vi "draw_field.vi"(0 "Field_Astrometry":T2 {"NAXIS" format="%#.6g"}, 1 "FOV":dbl, 2 "NaxisMax":dbl=1000000.0, 3 "Ring":u16(ring) items=["Square", "Circle"], 5 "Table_Astrometry":T2 {"CRPIX" format="%.1f"}, 6 "Rotation effective":dbl, 9 "Ues Constant Size ?":bool, 11 "margin/size":dbl=5.0, 12 "MirrorAvatar":T1={"Empreinte du miroir [arcmin]"=12.075, "Cur X"=-5.0, "Cur Y"=35.0, "Vignetting du miroir [armin]"=17.764, "FOV du miroir [arcmin]"=12.075, "LimXPesto"=-5.0, "BrasPesto"=FALSE}) -> (4 "TableXYPos":cluster{dbl[], dbl[]}[](graph), 10 "X Scale.Range":T3, 13 "ImgDEC":dbl format="%.6f", 14 "ImgRA":dbl format="%.6f", 15 "Y Scale.Range":T3)   [LabVIEW 2019]
uses:
  <vilib>/Utility/miscctls.llb/LVRangeTypeDef.ctl
  <vilib>/Analysis/coordinate.llb/2D Cartesian Coordinate Rotation (Array).vi
  <vilib>/Analysis/baseanly.llb/Mean (DBL).vi
  <vilib>/Analysis/NI_AALPro.lvlib
  <vilib>/Analysis/NI_AALBase.lvlib
panel:
  out "Rotation effective (rad)":dbl
  out "Vig Y":dbl[](array[numeric])
  out "Vig X":dbl[](array[numeric])
  in  "RayondeVignetting [arcmin]":dbl=50.0
  out "Y_arr":dbl[](array[numeric])
  out "X_arr":dbl[](array[numeric])
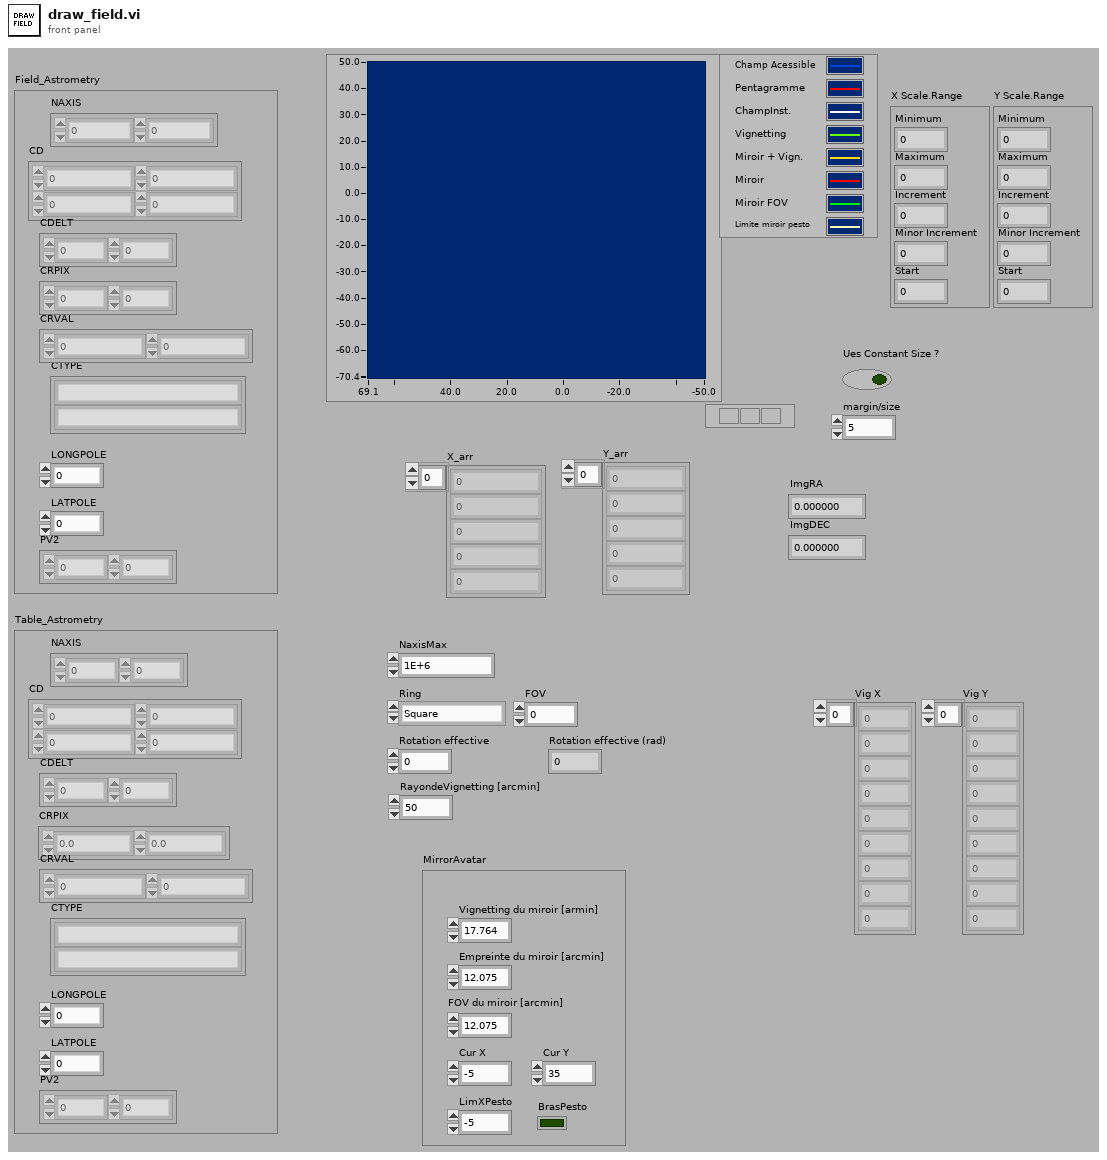
[diagram p1: front panel]
types:
  T1 = cluster{"Empreinte du miroir [arcmin]":dbl, "Cur X":dbl, "Cur Y":dbl, "Vignetting du miroir [armin]":dbl, "FOV du miroir [arcmin]":dbl, "LimXPesto":dbl, "BrasPesto":bool}
  T2 = cluster{"NAXIS":dbl[], "CD":dbl[][], "CDELT":dbl[], "CRPIX":dbl[], "CTYPE":string[], "CRVAL":dbl[], "LONGPOLE":dbl, "LATPOLE":dbl, "PV2":dbl[]}
  T3 = typedef "LVRangeTypeDef.ctl" = cluster{"Minimum":dbl, "Maximum":dbl, "Increment":dbl, "Minor Increment":dbl, "Start":dbl}
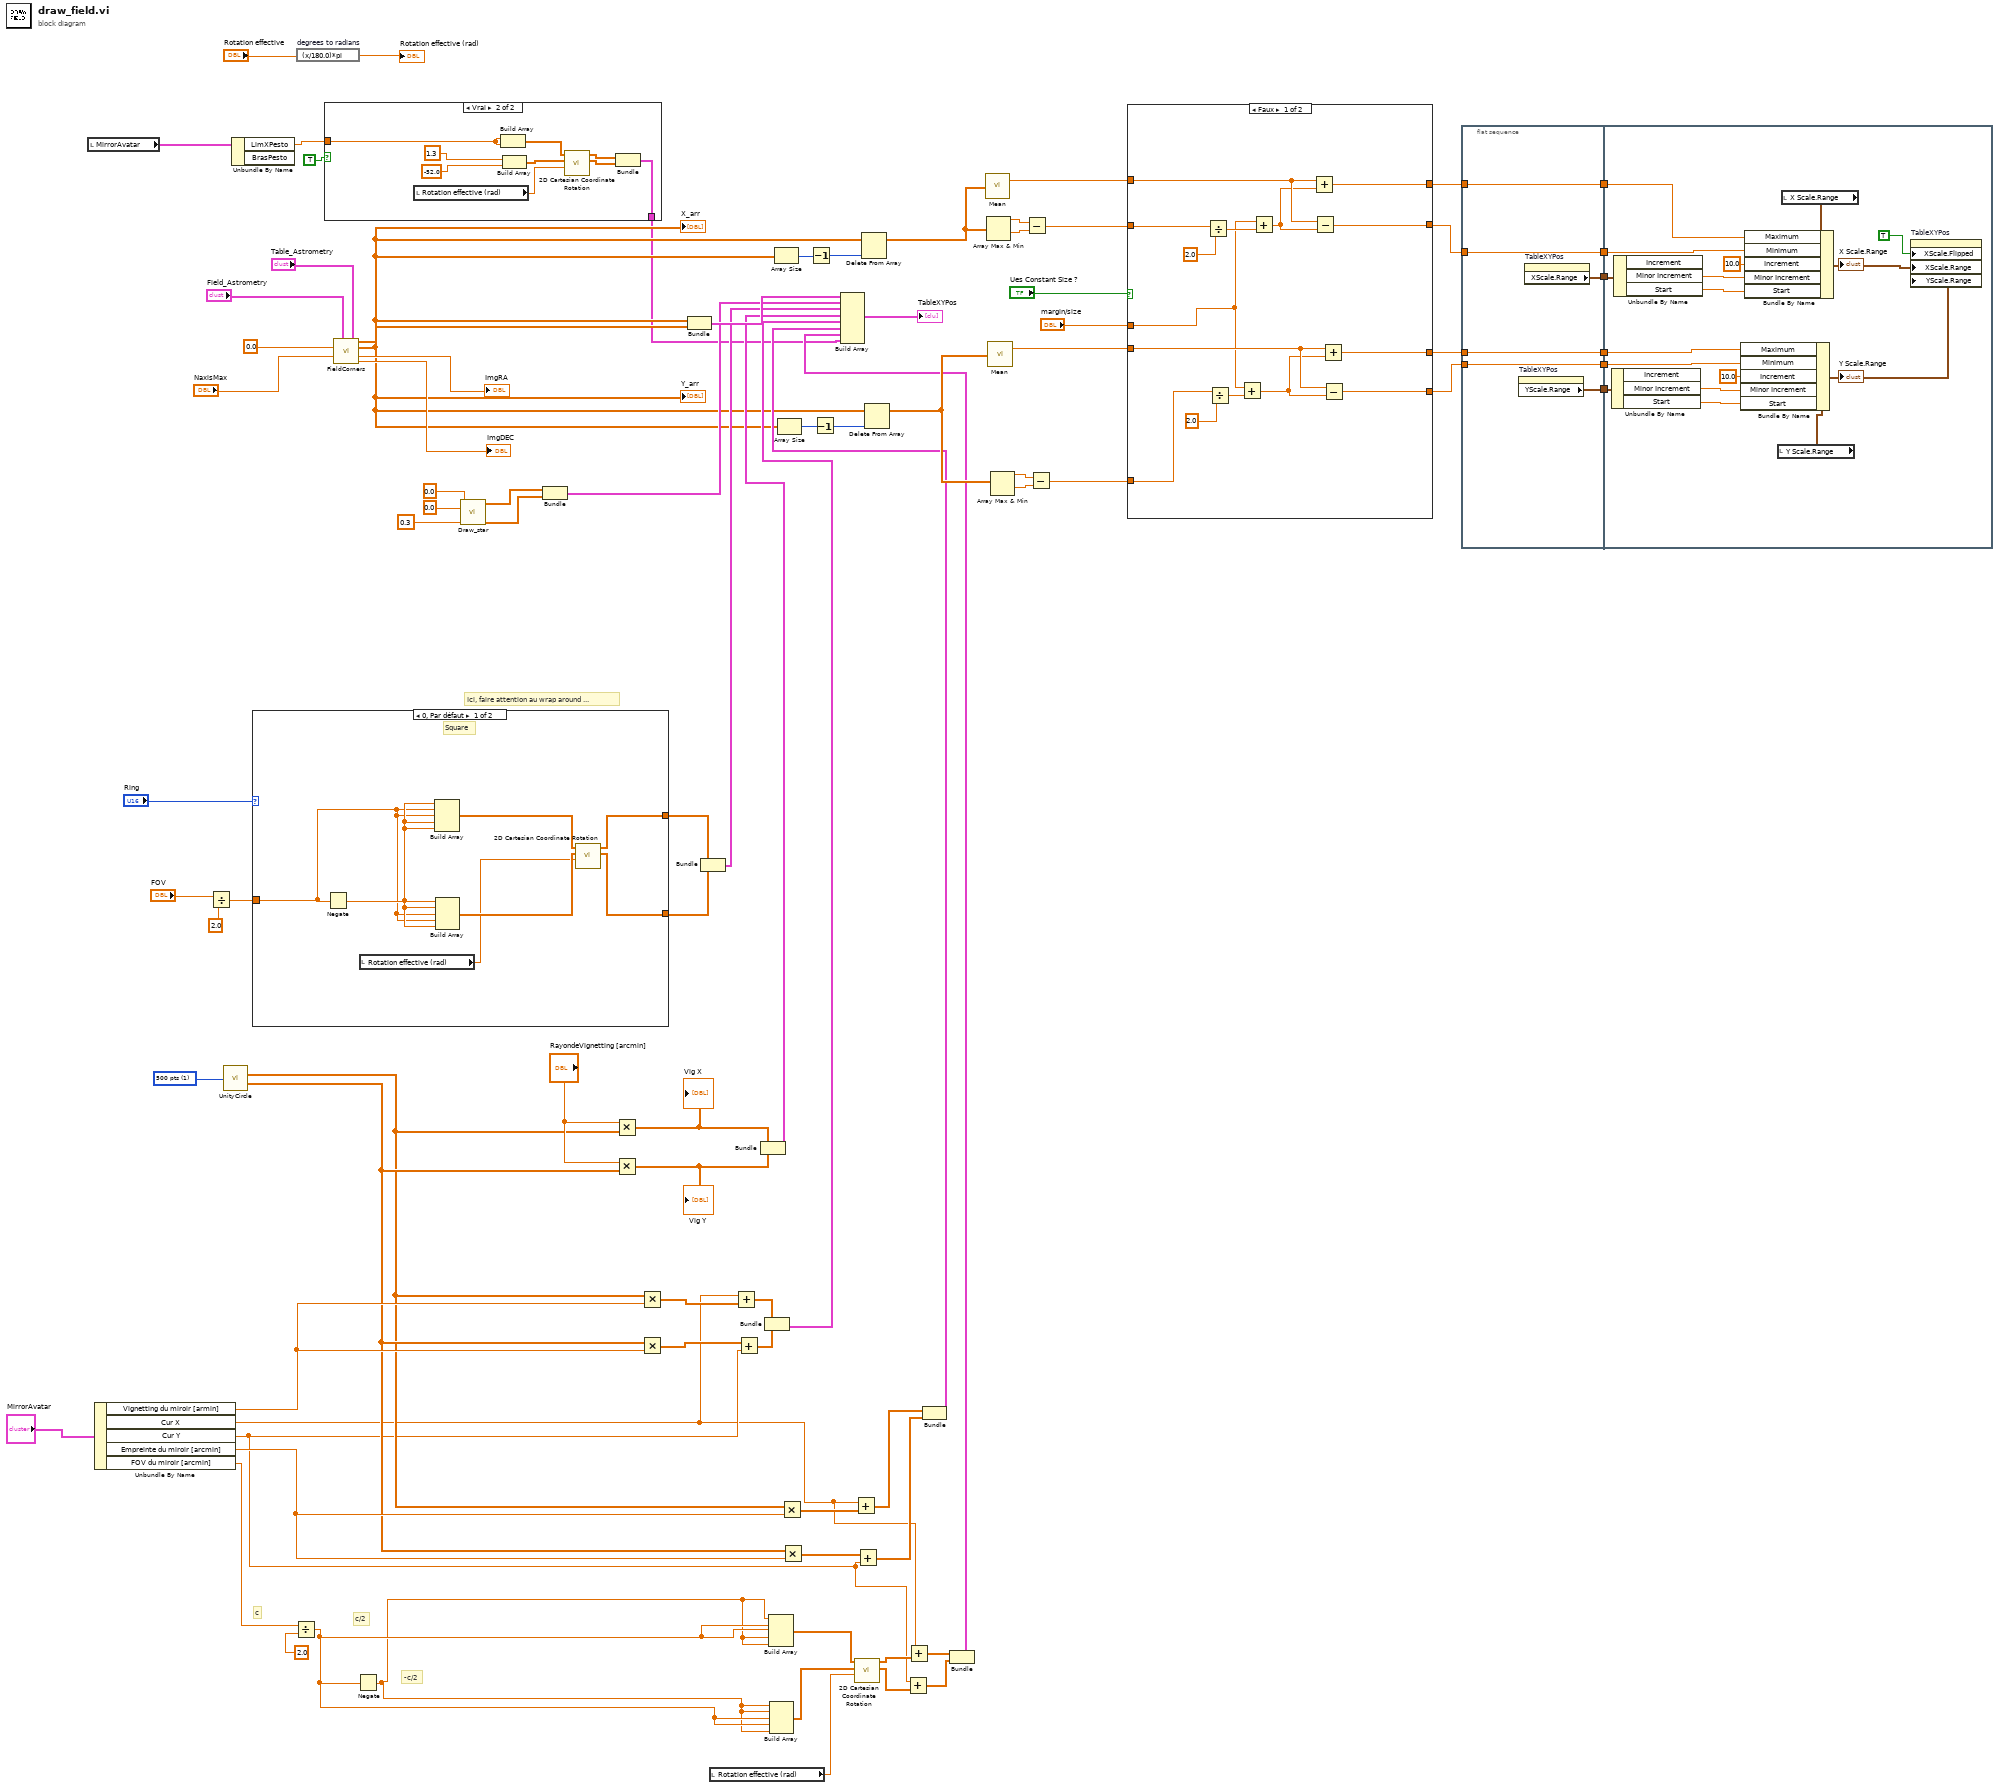
[diagram p0: block diagram]
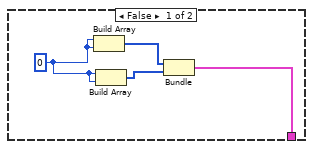
[diagram p2: hidden frame]
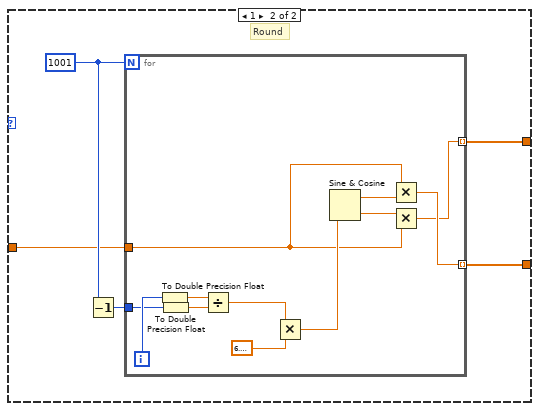
[diagram p3: hidden frame]
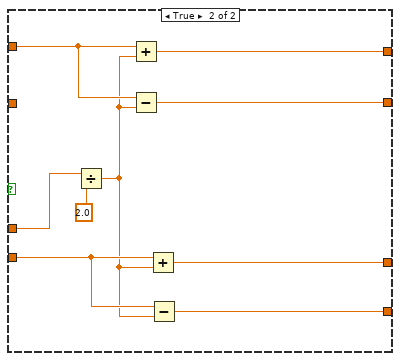
[diagram p4: hidden frame]
diagram:
  w30 = u16 1 items=["100 pts", "500 pts", "1000 pts"] ("Ring")
  # "c"
  # "c/2"
  # "-c/2"
  # "Ici, faire attention au wrap around ..."
  n1 = local read "MirrorAvatar"() -> (w3:T1)
  n2 = Unbundle By Name("MirrorAvatar") -> ("Vignetting du miroir [armin]"=w26:dbl, "Cur X"=w6:dbl, "Cur Y"=w7:dbl, "Empreinte du miroir [arcmin]"=w25:dbl, "FOV du miroir [arcmin]"=w21:dbl)
  n3 = Divide(x="FOV", y=2.0) -> (x/y=w60:dbl)
  n4 = call "UnityCircle.vi"("Ring"=w30) -> ("Circle X"=w23:dbl[], "Circle Y"=w24:dbl[])  [unwired: 13 in]
  n5 = Unbundle By Name(w3) -> ("LimXPesto"=w2:dbl)  [unwired: 1 out]
  n6 = case shown="0, Par défaut" "Ring" {
    tunnel: w60 -> [w95 w99]
    tunnel: [w91 w97] -> w65
    tunnel: [w90 w98] -> w64
    frame 0, Default {
      # "Square"
      n7 = Negate(x=w95) -> (-x=w96:dbl)
      n8 = local read "Rotation effective (rad)"() -> (w92:dbl)
      n9 = Build Array(w96, w95, w95, w96, w96) -> (w94:dbl[])
      n10 = Build Array(w96, w96, w95, w95, w96) -> (w93:dbl[])
      n11 = call-poly <vilib>:"2D Cartesian Coordinate Rotation.vi"("theta"=w92, "Y"=w93, "X"=w94) -> ("Y Out"=w90:dbl[], "X Out"=w91:dbl[])  [unwired: 6 in, 1 out]
    }
    frame 1 {
      w100 = 1001
      # "Round"
      n12 = Decrement(x=w100) -> (x-1=w101:i32)
      n13 = for {
        N: w100 -> [_]
        tunnel: w101 -> [w109]
        tunnel: w99 -> [w104]
        tunnel: [w103] -> w98 mode=indexing
        tunnel: [w102] -> w97 mode=indexing
        i -> [w113]
        n14 = To Double Precision Float(number=w113) -> (double precision float=w111:dbl)
        n15 = To Double Precision Float(number=w109) -> (double precision float=w110:dbl)
        n16 = Divide(x=w111, y=w110) -> (x/y=w108:dbl)
        n17 = Multiply(x=w108, y=6.283185307179586) -> (x*y=w107:dbl)
        n18 = Sine & Cosine(0:w107) -> (1:w106:dbl, 2:w105:dbl)
        n19 = Multiply(x=w104, y=w106) -> (x*y=w103:dbl)
        n20 = Multiply(x=w105, y=w104) -> (x*y=w102:dbl)
      }
    }
  }
  n21 = Divide(x=w21, y=2.0) -> (x/y=w11:dbl)
  n22 = expression code="(x/180.0)*pi" "degrees to radians"("Rotation effective") -> (→"Rotation effective (rad)":dbl)
  n23 = case shown="Vrai" TRUE {
    tunnel: [w114 w126] -> w17
    tunnel: w2 -> [_ w118]
    frame False {
      w117 = 0
      n24 = Build Array(w117, w117) -> (w116:i32[])
      n25 = Build Array(w117, w117) -> (w115:i32[])
      n26 = Bundle(w116, w115) -> (w114:cluster{i32[], i32[]})  [unwired: 1 in]
    }
    frame True {
      n27 = local read "Rotation effective (rad)"() -> (w119:dbl)
      n28 = Build Array(w118, w118) -> (w122:dbl[])
      n29 = Build Array(1.3 ("element"), -52.0 ("element")) -> (w123:dbl[])
      n30 = call-poly <vilib>:"2D Cartesian Coordinate Rotation.vi"("theta"=w119, "Y"=w123, "X"=w122) -> ("Y Out"=w124:dbl[], "X Out"=w125:dbl[])  [unwired: 6 in, 1 out]
      n31 = Bundle("X Out"=w125, "Y Out"=w124) -> (w126:cluster{"X Out":dbl[], "Y Out":dbl[]})  [unwired: 1 in]
    }
  }
  n32 = call "FieldCorners.vi"("Field_Astrometry"="Field_Astrometry", "Table_Astrometry"="Table_Astrometry", "NaxisMin"=0.0, "NaxisMax"="NaxisMax") -> ("X's"=w19:dbl[], "Y's"=w18:dbl[], "MeanRA"=→"ImgRA":dbl, "MeanDEC"=→"ImgDEC":dbl)  [unwired: 8 in]
  "X_arr" <- w19
  "Y_arr" <- w18
  n33 = Negate(x=w11) -> (-x=w10:dbl)
  n34 = call "Draw_star.vi"("size"=0.3, "DEC (°)"=0.0, "RA (°)"=0.0) -> ("Y"=w77:dbl[], "X"=w78:dbl[])  [unwired: 7 in]
  n35 = Bundle("X"=w78, "Y"=w77) -> (w80:cluster{"X":dbl[], "Y":dbl[]})  [unwired: 1 in]
  n36 = Multiply(x="RayondeVignetting [arcmin]", y=w23) -> (x*y=w29:dbl[])
  "Vig X" <- w29
  n37 = Multiply(x="RayondeVignetting [arcmin]", y=w24) -> (x*y=w28:dbl[])
  "Vig Y" <- w28
  n38 = Multiply(x=w23, y=w26) -> (x*y=w32:dbl[])
  n39 = Multiply(x=w24, y=w26) -> (x*y=w31:dbl[])
  n40 = Bundle("X's"=w19, "Y's"=w18) -> (w82:cluster{"X's":dbl[], "Y's":dbl[]})  [unwired: 1 in]
  n41 = Bundle("X Out"=w65, "Y Out"=w64) -> (w63:cluster{"X Out":dbl[], "Y Out":dbl[]})  [unwired: 1 in]
  n42 = local read "Rotation effective (rad)"() -> (w14:dbl)
  n43 = Add(x=w6, y=w32) -> (x+y=w41:dbl[])
  n44 = Add(x=w31, y=w7) -> (x+y=w40:dbl[])
  n45 = Bundle(w29, w28) -> (w42:cluster{dbl[], dbl[]})  [unwired: 1 in]
  n46 = Bundle(w41, w40) -> (w39:cluster{dbl[], dbl[]})  [unwired: 1 in]
  n47 = Build Array(w10, w11, w11, w10, w10) -> (w12:dbl[])
  n48 = Build Array(w10, w10, w11, w11, w10) -> (w13:dbl[])
  n49 = Array Size(array=w19) -> (size(s)=w68:i32)
  n50 = Array Size(array=w18) -> (size(s)=w71:i32)
  n51 = Multiply(x=w23, y=w25) -> (x*y=w35:dbl[])
  n52 = Multiply(x=w24, y=w25) -> (x*y=w36:dbl[])
  n53 = Decrement(x=w68) -> (x-1=w69:i32)
  n54 = Decrement(x=w71) -> (x-1=w70:i32)
  n55 = Add(x=w6, y=w35) -> (x+y=w34:dbl[])
  n56 = call-poly <vilib>:"2D Cartesian Coordinate Rotation.vi"("theta"=w14, "Y"=w13, "X"=w12) -> ("Y Out"=w8:dbl[], "X Out"=w9:dbl[])  [unwired: 6 in, 1 out]
  n57 = Add(x=w36, y=w7) -> (x+y=w33:dbl[])
  n58 = Delete From Array(array=w19, index=w69) -> (array with subset deleted=w66:dbl[])  [unwired: 1 in, 1 out]
  n59 = Delete From Array(array=w18, index=w70) -> (array with subset deleted=w67:dbl[])  [unwired: 1 in, 1 out]
  n60 = Add(x=w7, y=w8) -> (x+y=w4:dbl[])
  n61 = Add(x=w6, y=w9) -> (x+y=w5:dbl[])
  n62 = Bundle(w34, w33) -> (w37:cluster{dbl[], dbl[]})  [unwired: 1 in]
  n63 = Bundle(w5, w4) -> (w22:cluster{dbl[], dbl[]})  [unwired: 1 in]
  n64 = Build Array(w82, w80, w63, w42, w39, w37, w22, w17) -> (→"TableXYPos":cluster{"X Out":dbl[], "Y Out":dbl[]}[])
  n65 = call-poly <vilib>:"Mean.vi"("X"=w66) -> ("mean"=w73:dbl)  [unwired: 1 out]
  n66 = Array Max & Min(array=w66) -> (max value=w89:dbl, min value=w88:dbl)  [unwired: 2 out]
  n67 = call-poly <vilib>:"Mean.vi"("X"=w67) -> ("mean"=w72:dbl)  [unwired: 1 out]
  n68 = Array Max & Min(array=w67) -> (max value=w87:dbl, min value=w86:dbl)  [unwired: 2 out]
  n69 = Subtract(x=w89, y=w88) -> (x-y=w85:dbl)
  n70 = Subtract(x=w87, y=w86) -> (x-y=w76:dbl)
  n71 = case shown="Faux" "Ues Constant Size ?" {
    tunnel: w76 -> [w141 _]
    tunnel: [w139 w143] -> w55
    tunnel: w72 -> [w138 w144]
    tunnel: [w137 w148] -> w58
    tunnel: [w136 w147] -> w57
    tunnel: w73 -> [w135 w146]
    tunnel: w85 -> [w133 _]
    tunnel: [w128 w145] -> w56
    tunnel: "margin/size" -> [w127 w150]
    frame False {
      n72 = Divide(x=w133, y=2.0) -> (x/y=w132:dbl)
      n73 = Divide(x=w141, y=2.0) -> (x/y=w130:dbl)
      n74 = Add(x=w127, y=w130) -> (x+y=w129:dbl)
      n75 = Add(x=w127, y=w132) -> (x+y=w131:dbl)
      n76 = Add(x=w135, y=w131) -> (x+y=w137:dbl)
      n77 = Subtract(x=w135, y=w131) -> (x-y=w136:dbl)
      n78 = Add(x=w138, y=w129) -> (x+y=w128:dbl)
      n79 = Subtract(x=w138, y=w129) -> (x-y=w139:dbl)
    }
    frame True {
      n80 = Divide(x=w150, y=2.0) -> (x/y=w142:dbl)
      n81 = Add(x=w146, y=w142) -> (x+y=w148:dbl)
      n82 = Subtract(x=w146, y=w142) -> (x-y=w147:dbl)
      n83 = Add(x=w144, y=w142) -> (x+y=w145:dbl)
      n84 = Subtract(x=w144, y=w142) -> (x-y=w143:dbl)
    }
  }
  n85 = flat-sequence {
    tunnel: w55 -> [w153]
    tunnel: w56 -> [w154]
    tunnel: w57 -> [w155]
    tunnel: w58 -> [w156]
    tunnel: [w156] -> w54
    tunnel: [w155] -> w53
    tunnel: [w154] -> w52
    tunnel: [w153] -> w51
    tunnel: [w152] -> w50
    tunnel: [w151] -> w49
    tunnel: w54 -> [w173]
    tunnel: w53 -> [w172]
    tunnel: w52 -> [w171]
    tunnel: w51 -> [w170]
    tunnel: w50 -> [w164]
    tunnel: w49 -> [w160]
    frame #0 {
      n86 = property on="TableXYPos" class="GraphXY (strict)"() -> ("YScale.Range"=w151:T3)  [unwired: 2 in, 2 out]
      n87 = property on="TableXYPos" class="GraphXY (strict)"() -> ("XScale.Range"=w152:T3)  [unwired: 2 in, 2 out]
    }
    frame #1 {
      n88 = Unbundle By Name(w160) -> ("Minor Increment"=w159:dbl, "Start"=w161:dbl)  [unwired: 1 out]
      n89 = Unbundle By Name(w164) -> ("Minor Increment"=w163:dbl, "Start"=w162:dbl)  [unwired: 1 out]
      n90 = local read "Y Scale.Range"() -> (w168:T3)
      n91 = Bundle By Name(cluster=w168, "Maximum"=w171, "Minimum"=w170, "Increment"=10.0, "Minor Increment"=w159, "Start"=w161) -> (w166:T3)
      "Y Scale.Range" <- w166
      n92 = local read "X Scale.Range"() -> (w169:T3)
      n93 = Bundle By Name(cluster=w169, "Maximum"=w173, "Minimum"=w172, "Increment"=10.0, "Minor Increment"=w163, "Start"=w162) -> (w167:T3)
      "X Scale.Range" <- w167
      n94 = property on="TableXYPos" class="GraphXY (strict)"("XScale.Flipped"=TRUE ("X Scale.Flipped"), "XScale.Range"=w167, "YScale.Range"=w166) -> ()  [unwired: 2 in, 2 out]
    }
  }
